vi "Get Data Variant.vi"(8 "error in (no error)":errorcluster, 11 "Core Channels Configuration in":refnum<class "Core Channel Configuration.lvclass">) -> (0 "error out":errorcluster, 1 "data version":T1, 2 "data":variant, 3 "Core Channels Configuration out":refnum<class "Core Channel Configuration.lvclass">)   [LabVIEW 2017, in "DSF Core.lvlib" / "Core Channel Configuration.lvclass"]
uses:
  Core Channel Configuration.lvclass
  Typedefs/DSF Version Info.ctl
  Core Channel Configuration.lvclass/Core Channel Configuration.ctl
  DSF Core.lvlib
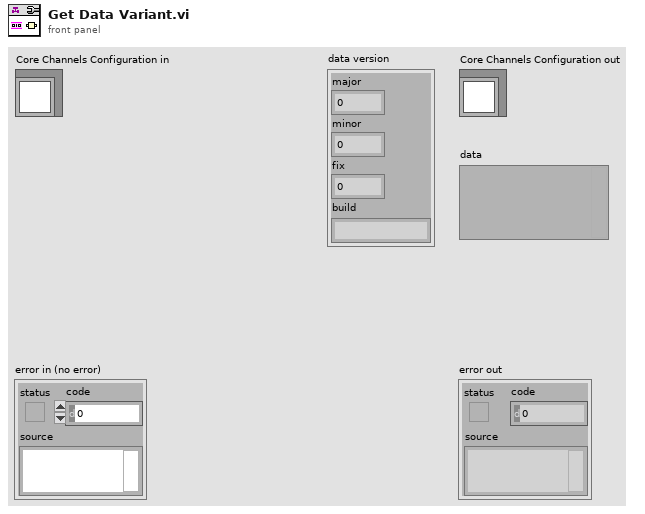
[diagram p1: front panel]
types:
  T1 = typedef "DSF Core.lvlib/DSF Version Info.ctl" = cluster{"major":u32, "minor":u32, "fix":u32, "build":string}
  T2 = typedef "DSF Core.lvlib/DSF Core Channel Configuration.ctl" = cluster{"name":string, "units":string, "engine data type":T3, "string data type":T3, "string offset":u64}
  T3 = typedef "DSF Core.lvlib/DSF Data Type.ctl" = enum8{"Bool", "SGL", "DBL", "I8", "I16", "I32", "I64", "U8", "U16", "U32", "U64"}
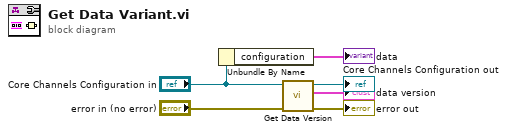
[diagram p0: block diagram]
diagram:
  n1 = Unbundle By Name("Core Channels Configuration in") -> ("configuration"=→"data":T2)
  n2 = call-dynamic "Get Data Version.vi"("error in (no error)"="error in (no error)", "Core Channels Configuration in"="Core Channels Configuration in") -> ("error out"=→"error out":errorcluster, "data version"=→"data version":T1, "Core Channels Configuration out"=→"Core Channels Configuration out":refnum<class "Core Channel Configuration.lvclass">)  [unwired: 7 in]
